vi "Read (Single Point).vi"(0 "VISA resource name":refnum<visa-resource-name>, 5 "Timeout (10000 ms)":i32=10000 format="%#.6g", 7 "Buffer Name (defbuffer1)":string="defbuffer1", 9 "Buffer Elements":string="READ", 11 "error in (no error)":errorcluster) -> (4 "VISA resource name out":refnum<visa-resource-name>, 6 "Data out":string, 15 "error out":errorcluster)   [LabVIEW 2017, in "Keithley 2450.lvlib"]
doc: "Reads and returns a single measurement from the instrument.\n\nBuffer Element can be a single parameter or multiple parameters.Parameters have to be separated by comma followed by space.(eg - READ, SEC, DATE)\n\n<B>Note:</B> Using this VI will overwrite all triggering settings with settings for a single point taken immediately. For control over the trigger, use the Low Level API."
uses:
  Keithley 2450.lvlib
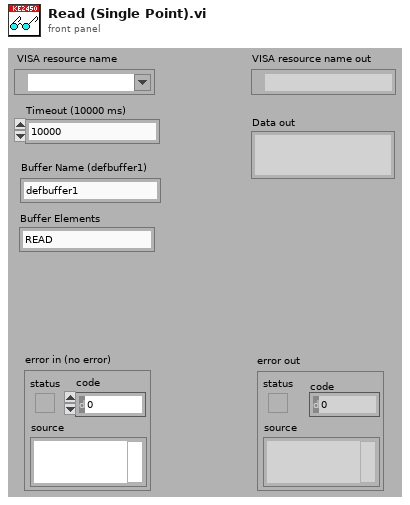
[diagram p1: front panel]
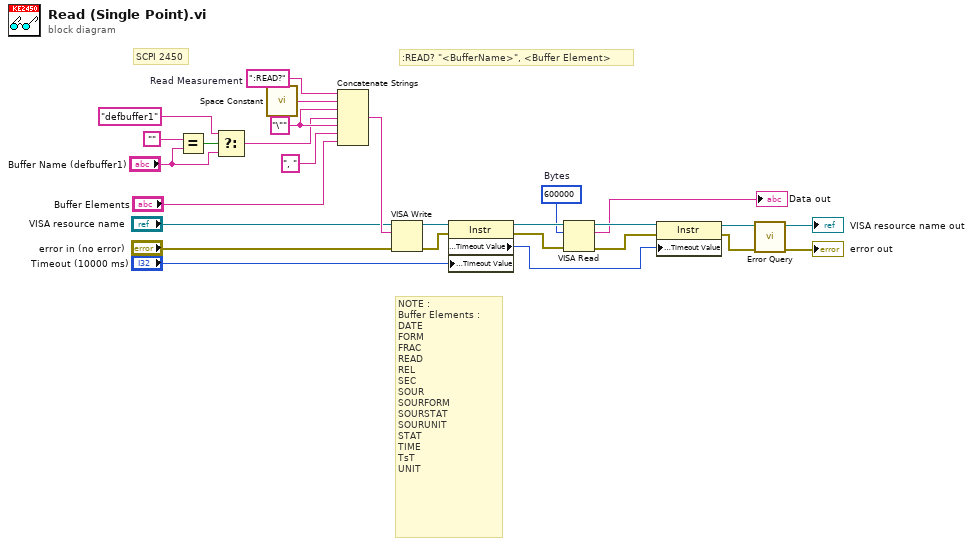
[diagram p0: block diagram]
diagram:
  w12 = "\""
  w9 = ":READ?"  # Read Measurement
  w19 = u32 600000  # Bytes
  # "NOTE :\nBuffer Elements :\nDATE\nFORM\nFRAC\nREAD\nREL\nSEC\nSOUR\nSOURFORM\nSOURSTAT\nSOURUNIT\nSTAT\nTIME\nTsT\nUNIT"
  # ":READ? \"<BufferName>\", <Buffer Element>"
  # "SCPI 2450"
  n1 = Equal?(x="", y="Buffer Name (defbuffer1)") -> (x = y?=w15:bool)
  n2 = Select(t="defbuffer1", s=w15, f="Buffer Name (defbuffer1)") -> (s? t:f=w11:string)
  n3 = call <vilib>:"Space Constant.vi"() -> ("String"=w10:string)
  n4 = Concatenate Strings(w9, w10, w12, w11, w12, ", " ("string"), "Buffer Elements") -> (w26:string)
  n5 = VISA Write(VISA resource name="VISA resource name", write buffer=w26, error in (no error)="error in (no error)") -> (VISA resource name out=w17:refnum<visa-resource-name>, error out=w25:errorcluster)  [unwired: 1 out]
  n6 = property class="Instr"(reference=w17, error in=w25, "General Settings:Timeout Value"="Timeout (10000 ms)") -> (reference out=w24:refnum<visa-resource-name>, error out=w23:errorcluster, "General Settings:Timeout Value"=w20:u32)
  n7 = VISA Read(VISA resource name=w24, byte count=w19, error in (no error)=w23) -> (VISA resource name out=w22:refnum<visa-resource-name>, read buffer=→"Data out":string, error out=w21:errorcluster)  [unwired: 1 out]
  n8 = property class="Instr"(reference=w22, error in=w21, "General Settings:Timeout Value"=w20) -> (reference out=w5:refnum<visa-resource-name>, error out=w4:errorcluster)
  n9 = call "Error Query.vi"("error in (no error)"=w4, "VISA resource name"=w5) -> ("error out"=→"error out":errorcluster, "VISA resource name out"=→"VISA resource name out":refnum<visa-resource-name>)  [unwired: 8 out]
